vi "Display Console View.vi"(8 "error in (no error)":errorcluster, 11 "View Model":T2) -> (0 "error out":errorcluster)   [LabVIEW 2017]
doc: "The interface where a user receives status updates from the Controller.\n[Covers: UI3]"
uses:
  View Model/Controls/View Model.ctl
  View Model/Controls/Shared Model.ctl
  Error/Controls/Error Model.ctl
  Error/Controls/Error Event.ctl
  Error/Controls/Error Type.ctl
  Configuration/Controls/Config DB Model.ctl
  Configuration/Controls/Config DB Command.ctl
  Configuration/Controls/Config DB Record.ctl
  Controller/Controls/Controller Model.ctl
  Controller/Controls/Elevator Location.ctl
  Controller/Controls/Elevator Direction Event.ctl
  Controller/Controls/Elevator Direction.ctl
panel:
  out "Emergency":bool
  out "Door Open":bool
  out "Down":bool
  out "Up":bool
  out "Elevator Location":T1
  out "Timing":dbl
  # "Elevator Direction"
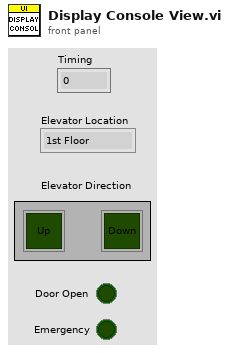
[diagram p1: front panel]
types:
  T1 = typedef "Elevator Location.ctl" = enum16{"1st Floor", "2nd Floor", "3rd Floor", "4th Floor"}
  T2 = typedef "View Model.ctl" = cluster{"Shared Model":T3, "Error Model":T4, "Config Model":T5, "Controller Model":T6}
  T3 = typedef "Shared Model.ctl" = cluster{"Stop":refnum<user-event>, "Stop DVR":refnum<data-value>}
  T4 = typedef "Error Model.ctl" = cluster{"Error":refnum<user-event>}
  T5 = typedef "Config DB Model.ctl" = cluster{"DB Command":refnum<user-event>, "DB Record DVR":refnum<data-value>}
  T6 = typedef "Controller Model.ctl" = cluster{"Go to Floor":refnum<user-event>, "Emergency":refnum<user-event>, "Open/Close Door":refnum<user-event>, "Move To":refnum<user-event>, "Position Change":refnum<user-event>}
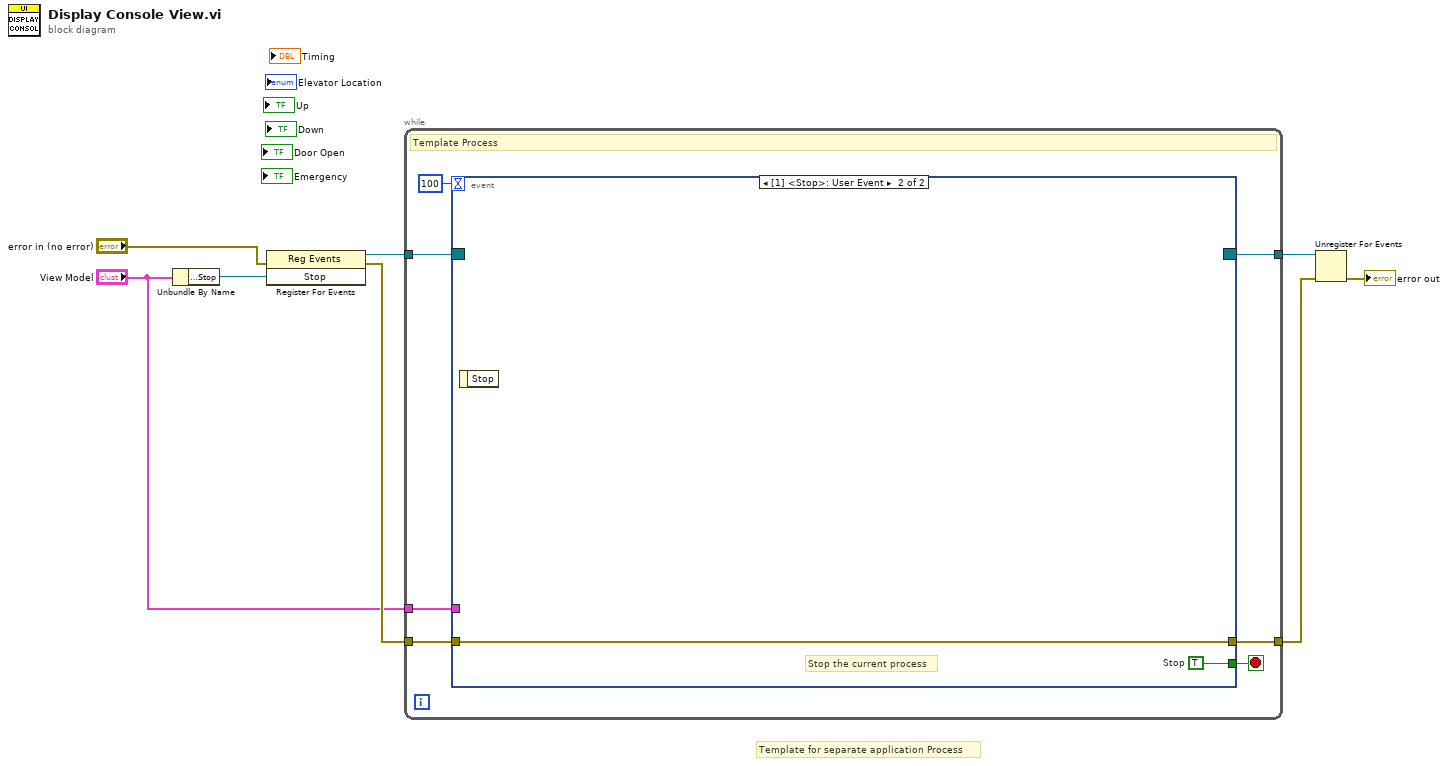
[diagram p0: block diagram]
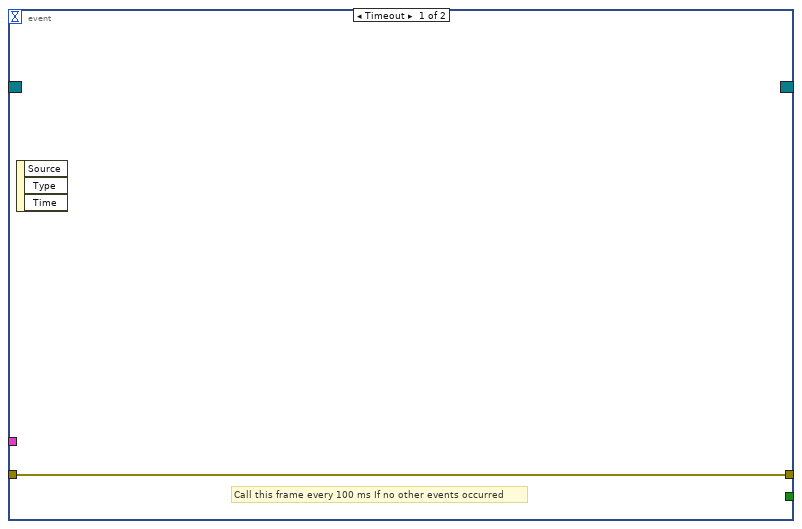
[diagram p2: hidden frame]
diagram:
  # "Template for separate application Process"
  n1 = Unbundle By Name("View Model") -> ("Shared Model.Stop"=w8:refnum<user-event>)
  n2 = register-events(error in="error in (no error)", w8) -> (reference out=w7:refnum<event-registration>, error out=w4:errorcluster)  [unwired: 1 in]
  n3 = while {
    tunnel: w7 -> [w15]
    tunnel: [w14] -> w6
    tunnel: w4 -> [w13]
    tunnel: "View Model" -> [w12]
    tunnel: [w11] -> w2
    stop <- w10 stop-if-true
    # "Template Process"
    n4 = event shown="[1] <Stop>: User Event" {
      selector: w15 -> [_ _]
      dyn-events: [_ _] -> w14
      timeout: 100 -> [_ _]
      tunnel: w13 -> [w16 w18]
      tunnel: w12 -> [_ _]
      tunnel: [w16 w18] -> w11
      tunnel: [_ w17] -> w10
      event Timeout {
        # "Call this frame every 100 ms If no other events occurred"
        n5 = event-data() -> ()  [unwired: 1 in, 3 out]
      }
      event User Event {
        w17 = TRUE  # Stop
        # "Stop the current process"
        n6 = event-data() -> ()  [unwired: 1 in, 1 out]
      }
    }
  }
  n7 = Unregister For Events(event registration refnum=w6, error in=w2) -> (error out=→"error out":errorcluster)
